vi "Run.vi"(8 "error in (no error)":errorcluster, 11 "Replay in":refnum<class "Replay.lvclass">) -> (0 "error out":errorcluster, 3 "Replay out":refnum<class "Replay.lvclass">)   [LabVIEW 2016, in "CLD Exam - ATM.lvlib" / "Replay.lvclass"]
uses:
  Replay.lvclass
  D:/Repos/Stream/software/Mediator/Classes/Mediated Actor/Mediated Actor.lvclass
  Mediator/Classes/Message Interface/Message Interface.lvclass
  Replay.lvclass/Replay.ctl
  Mediator/Classes/Message String/Message String.lvclass
  D:/Repos/Stream/software/Mediator/Classes/Message Interface/Message Interface.lvclass
  Mediator/Classes/Message Transport Queue/Message Transport Queue.lvclass
  Mediator/Classes/Mediated Actor/Mediated Actor.lvclass
panel:
  in  "Playback":bool
  in  "Event Log Path":path
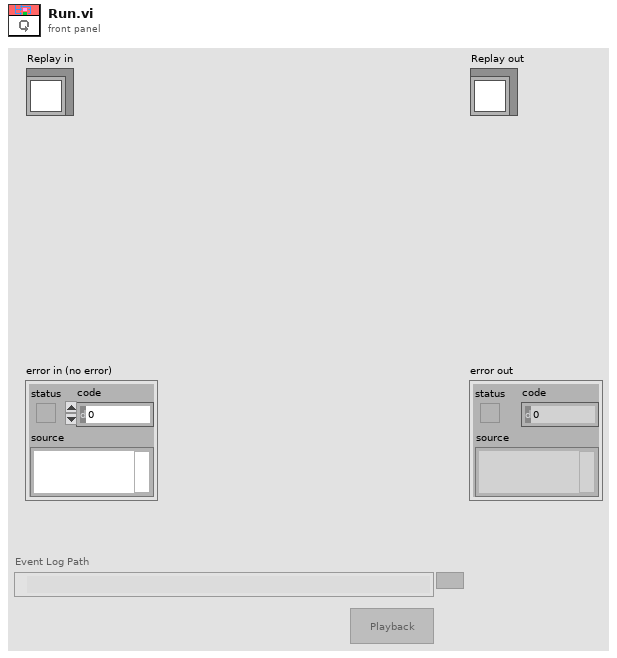
[diagram p1: front panel]
types:
  T1 = cluster{"System Exit":refnum<event-registration>, "To Self":refnum<event-registration>}
  T2 = enum8{"Enabled", "Disabled", "Disabled and Grayed Out"}
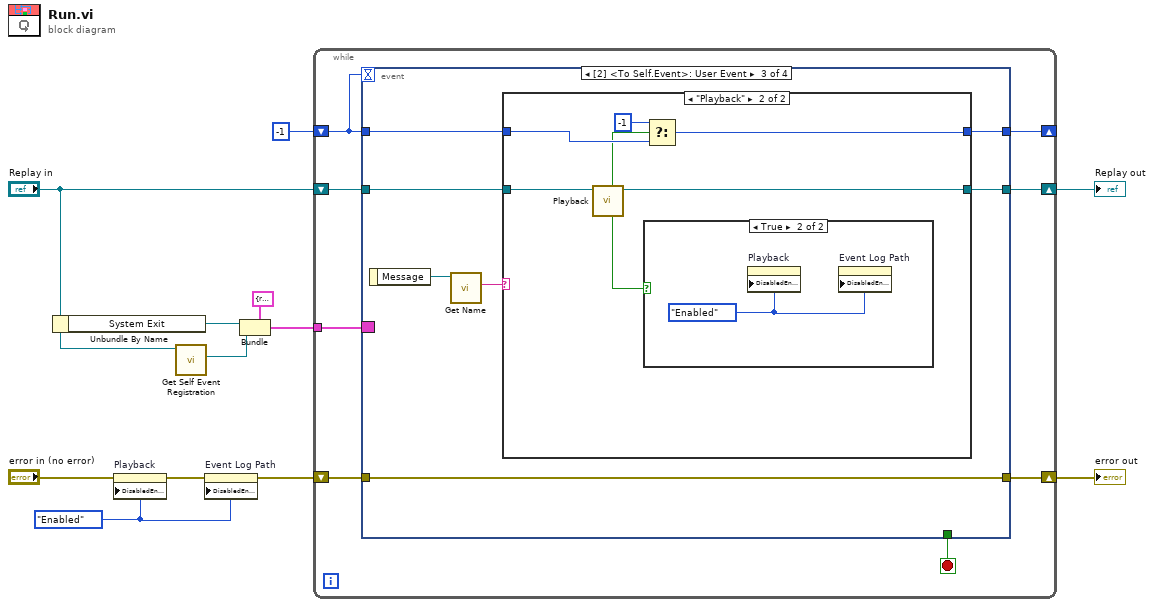
[diagram p0: block diagram]
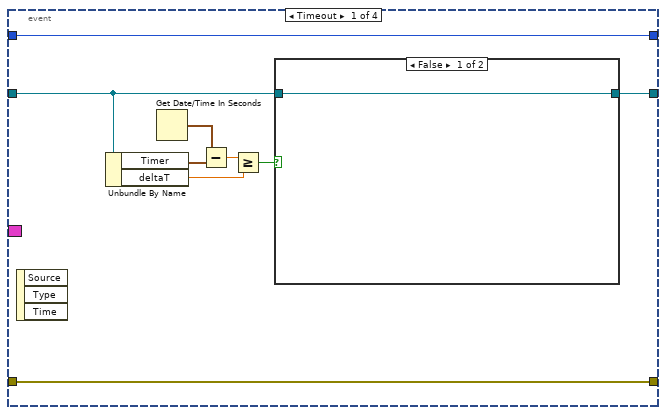
[diagram p2: hidden frame]
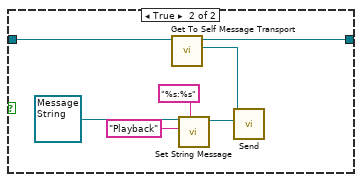
[diagram p3: hidden frame]
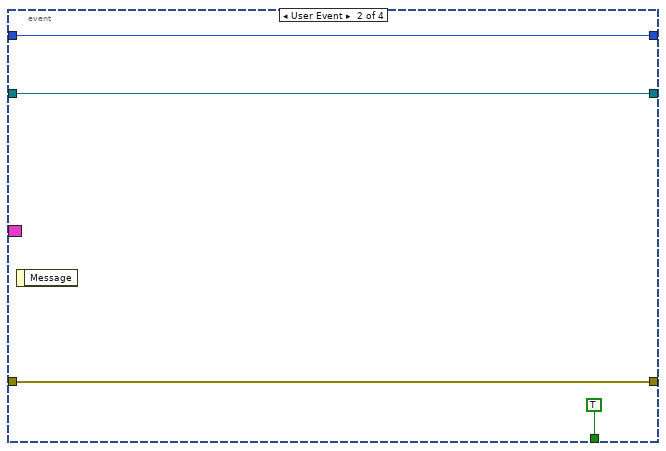
[diagram p4: hidden frame]
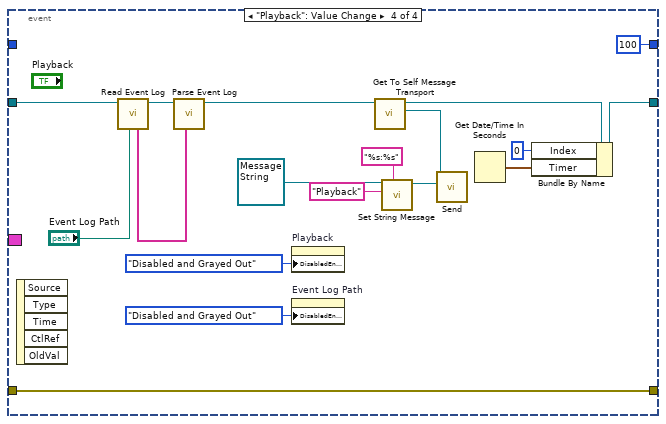
[diagram p7: hidden frame]
diagram:
  w2 = T2."Enabled" ("Disabled")
  n1 = Unbundle By Name("Replay in") -> ("System Exit"=w10:refnum<event-registration>)
  n2 = property on="Playback" class="Bool"(error in="error in (no error)", "DisabledEnum"=w2) -> (error out=w4:errorcluster)  [unwired: 1 in, 1 out]
  n3 = call "Get Self Event Registration.vi"("Mediated Actor in"="Replay in") -> ("Event Registration Refnum"=w9:refnum<event-registration>)  [unwired: 9 in, 1 out]
  n4 = property on="Event Log Path" class="Path"(error in=w4, "DisabledEnum"=w2) -> (error out=w3:errorcluster)  [unwired: 1 in, 1 out]
  n5 = Bundle(cluster=T1 {"System Exit"=refnum, "To Self"=refnum}, "System Exit"=w10, "To Self"=w9) -> (w8:T1)
  n6 = while {
    shift-right: [w19] -> w12
    shift-left: "Replay in" -> [w20]
    tunnel: w8 -> [w18]
    shift-right: [w15] -> w7
    shift-left: w3 -> [w16]
    shift-right: [w13] -> _
    shift-left: -1 -> [w14]
    stop <- w17 stop-if-true
    n7 = event shown="[2] <To Self.Event>: User Event" {
      selector: w18 -> [_ _ _ _]
      dyn-events: _ -> [_ _ _ _]
      timeout: w14 -> [_ _ _ _]
      tunnel: w20 -> [w23 w41 w45 w74]
      tunnel: [w22 w41 w44 w62] -> w19
      tunnel: [_ TRUE _ _] -> w17
      tunnel: w16 -> [w29 w39 w48 w75]
      tunnel: [w29 w39 w48 w75] -> w15
      tunnel: w14 -> [w28 w38 w43 _]
      tunnel: [w28 w38 w42 100] -> w13
      event Timeout {
        n8 = event-data() -> ()  [unwired: 1 in, 3 out]
        n9 = Unbundle By Name(w23) -> ("Timer"=w27:timestamp, "deltaT"=w24:dbl)
        n10 = Get Date/Time In Seconds() -> (seconds since 1Jan1904=w26:timestamp)
        n11 = Subtract(x=w26, y=w27) -> (x-y=w25:dbl)
        n12 = Greater Or Equal?(x=w25, y=w24) -> (x >= y?=w21:bool)
        n13 = case shown="False" w21 {
          tunnel: w23 -> [w30 w32]
          tunnel: [w30 w31] -> w22
          frame False {
          }
          frame True {
            n14 = call "Get To Self Message Transport.vi"("Mediated Actor in"=w32) -> ("To Self"=w35:refnum<class "Message Transport Queue.lvclass">, "Mediated Actor out"=w31:refnum<class "Replay.lvclass">)  [unwired: 9 in]
            n15 = call "Set String Message.vi"("Format"="%s:%s", "Name"="Playback", "Message String in"=refnum<class "Message String.lvclass"> refnum) -> ("Message String out"=w34:refnum<class "Message String.lvclass">)  [unwired: 7 in, 1 out]
            n16 = call-dynamic "Send.vi"("Message"=w34, "Message Transport Queue in"=w35) -> ()  [unwired: 7 in, 3 out]
          }
        }
      }
      event User Event {
        n17 = event-data() -> ()  [unwired: 1 in, 1 out]
      }
      event User Event {
        n18 = event-data() -> ("Message"=w47:refnum<class "Message Interface.lvclass">)  [unwired: 1 in]
        n19 = call "Get Name.vi"("Message Interface in"=w47) -> ("Name"=w46:string)  [unwired: 8 in, 2 out]
        n20 = case shown="\"Playback\"" w46 {
          tunnel: [w50 w55] -> w44
          tunnel: w45 -> [w50 w56]
          tunnel: [w49 w52] -> w42
          tunnel: w43 -> [w49 w53]
          frame Default {
          }
          frame "Playback" {
            n21 = call "Playback.vi"("Replay in"=w56) -> ("Replay out"=w55:refnum<class "Replay.lvclass">, "Done?"=w51:bool)  [unwired: 8 in, 1 out]
            n22 = case shown="True" w51 {
              frame False {
              }
              frame True {
                w57 = T2."Enabled" ("Disabled")
                n23 = property on="Playback" class="Bool"("DisabledEnum"=w57) -> ()  [unwired: 2 in, 2 out]
                n24 = property on="Event Log Path" class="Path"("DisabledEnum"=w57) -> ()  [unwired: 2 in, 2 out]
              }
            }
            n25 = Select(t=-1, s=w51, f=w53) -> (s? t:f=w52:i32)
          }
        }
      }
      event "Playback": Value Change {
        n26 = event-data() -> ()  [unwired: 1 in, 5 out]
        n27 = call "Read Event Log.vi"("Event Log Path"="Event Log Path", "Replay in"=w74) -> ("Replay out"=w72:refnum<class "Replay.lvclass">, "Log Data"=w71:string[])  [unwired: 7 in, 1 out]
        n28 = call "Parse Event Log.vi"("Log Data"=w71, "Replay in"=w72) -> ("Replay out"=w67:refnum<class "Replay.lvclass">)  [unwired: 8 in, 1 out]
        n29 = property on="Playback" class="Bool"("DisabledEnum"=T2."Disabled and Grayed Out" ("Disabled")) -> ()  [unwired: 2 in, 2 out]
        n30 = property on="Event Log Path" class="Path"("DisabledEnum"=T2."Disabled and Grayed Out" ("Disabled")) -> ()  [unwired: 2 in, 2 out]
        n31 = call "Get To Self Message Transport.vi"("Mediated Actor in"=w67) -> ("To Self"=w66:refnum<class "Message Transport Queue.lvclass">, "Mediated Actor out"=w63:refnum<class "Replay.lvclass">)  [unwired: 9 in]
        n32 = call "Set String Message.vi"("Format"="%s:%s", "Name"="Playback", "Message String in"=refnum<class "Message String.lvclass"> refnum) -> ("Message String out"=w65:refnum<class "Message String.lvclass">)  [unwired: 7 in, 1 out]
        n33 = call-dynamic "Send.vi"("Message"=w65, "Message Transport Queue in"=w66) -> ()  [unwired: 7 in, 3 out]
        n34 = Get Date/Time In Seconds() -> (seconds since 1Jan1904=w58:timestamp)
        n35 = Bundle By Name(cluster=w63, "Index"=u32 0 ("Data.Index"), "Timer"=w58) -> (w62:refnum<class "Replay.lvclass">)
      }
    }
  }
  "error out" <- w7
  "Replay out" <- w12
